vi "Autonomous Independent.vi"   [LabVIEW 2011]
doc: "This VI is called when autonomous begins, and will automatically be terminated when autonomous ends. You can carry out timed or sensor driven robot movement independently without needing to return to the caller."
uses:
  Robot Global Data.vi
types:
  T1 = typedef "WPI_MotorControlDeviceRef.ctl" = cluster{"DeviceStatus":errorcluster, "Type":enum16{"PWM", "CAN"}, "PWM":cluster{"Digital Module":T2, "PWM Channel":T3, "DeadBand":T4}, "CAN":cluster{"Device Number":u8, "Control Mode":T5, "Semaphore":T6, "Max Vout":dbl}, "Invert":bool, "TransformRef":T7, "InvTransformRef":T7}
  T2 = typedef "FPGA_TypedefDigitalModule.ctl" = enum16{"Digital Module 1", "Digital Module 2"}
  T3 = typedef "FPGA_DIOPWMChannel.ctl" = enum8{"PWM 1", "PWM 2", "PWM 3", "PWM 4", "PWM 5", "PWM 6", "PWM 7", "PWM 8", "PWM 9", "PWM 10", "Invalid"}
  T4 = typedef "WPI_PWMDeadband.ctl" = cluster{"Name":string, "maxPositivePwm":i32, "minPositivePwm":i32, "centerPwm":i32, "maxNegativePwm":i32, "minNegativePwm":i32, "angularRange":u16}
  T5 = typedef "WPI_CANJaguar_ControlMode.ctl" = enum8{"Percent VBus", "Current", "Speed", "Position", "Voltage"}
  T6 = typedef "Semaphore RefNum" = refnum<k1>
  T7 = typedef "WPI_PWMTransform_ConPane.ctl" = refnum<vi>
  T8 = typedef "WPI_ServoDeviceRef.ctl" = cluster{"DeviceStatus":errorcluster, "Digital Module":T2, "PWM Channel":T3, "DeadBand":T4}
  T9 = typedef "WPI_EncoderDevRef.ctl" = cluster{"DevStatus":errorcluster, "EncoderIndex":T10, "CounterIndex":T11, "DistancePerCount":dbl, "Decoding Type":T12}
  T10 = typedef "FPGA_EncoderIdx.ctl" = enum8{"Enc 0", "Enc 1", "Enc 2", "Enc 3", "Invalid"}
  T11 = typedef "FPGA_CounterCtrSystemIndex.ctl" = enum8{"Ctr 0", "Ctr 1", "Ctr 2", "Ctr 3", "Ctr 4", "Ctr 5", "Ctr 6", "Ctr 7", "Invalid"}
  T12 = typedef "WPI_EncoderType.ctl" = enum16{"1x", "2x", "4x"}
  T13 = typedef "WPI_GyroDevRef.ctl" = cluster{"DevStatus":errorcluster, "Analog Module":T14, "Analog Channel":T15, "Offset":dbl, "Gain (VoltsPerDegree/Second)":dbl}
  T14 = typedef "FPGA_TypedefAnalogModule.ctl" = enum16{"Analog Module 1", "Analog Module 2"}
  T15 = typedef "FPGA_AIChannel.ctl" = enum8{"AI 1", "AI 2", "AI 3", "AI 4", "AI 5", "AI 6", "AI 7", "AI 8", "Invalid"}
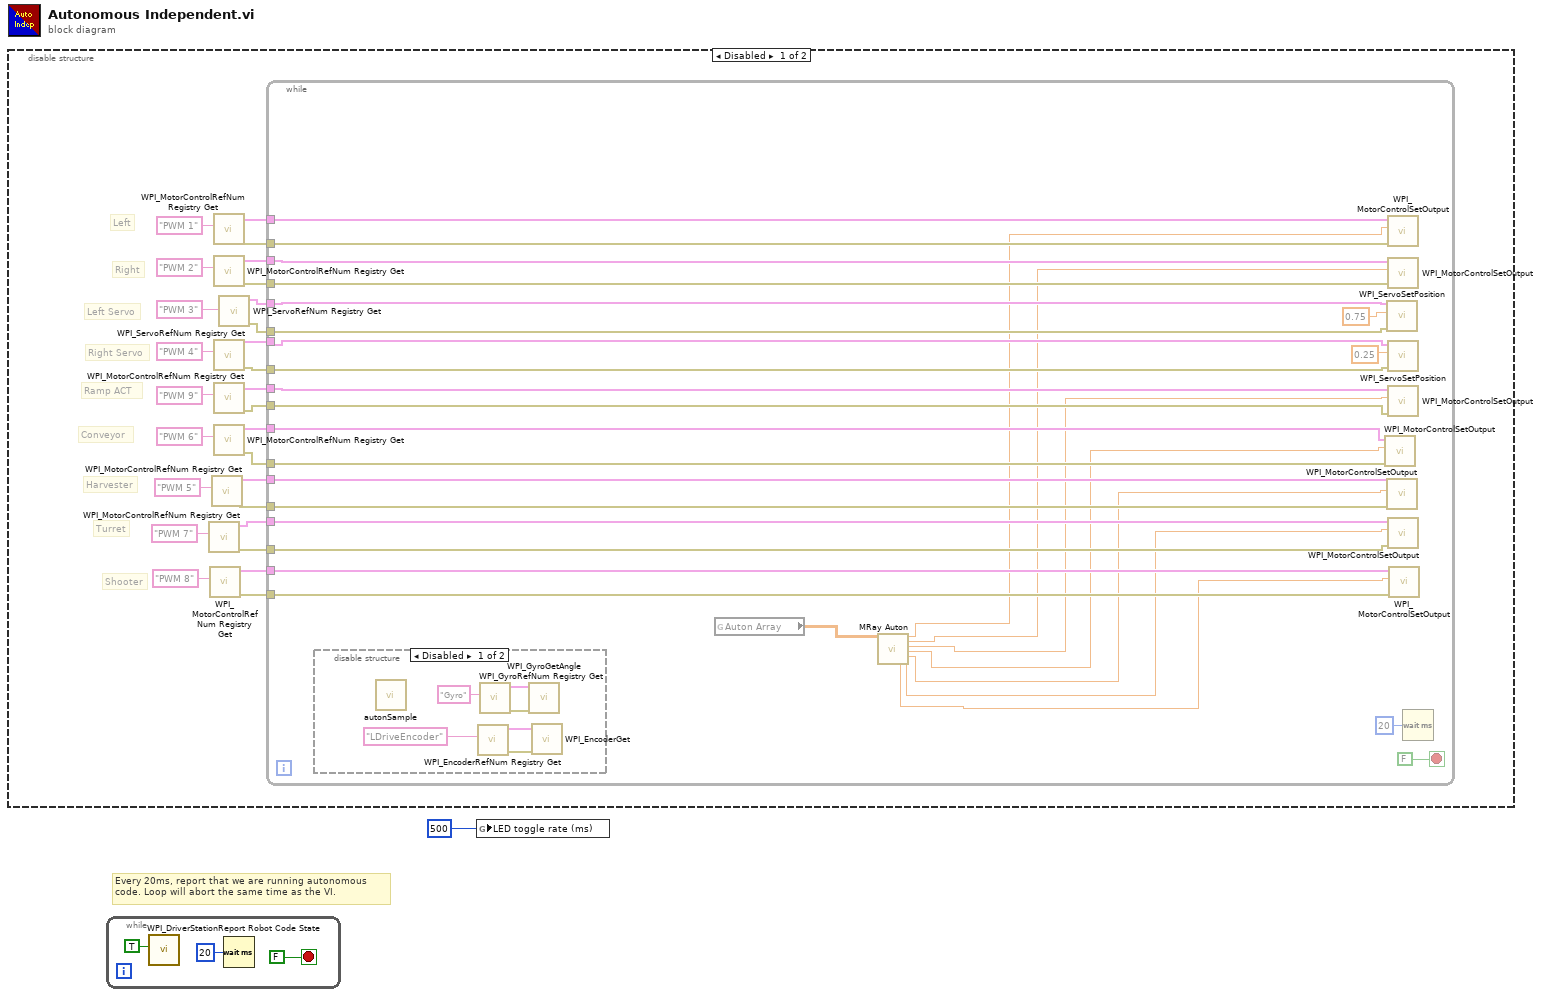
[diagram p0: block diagram]
diagram:
  # "Every 20ms, report that we are running autonomous\ncode. Loop will abort the same time as the VI."
  n1 = disable-structure shown="Disabled" {
    frame Disabled {
      # "Shooter"
      # "Turret"
      # "Conveyor"
      # "Harvester"
      # "Ramp ACT"
      # "Right Servo"
      # "Left Servo"
      # "Right"
      # "Left"
      n2 = call <vilib>:"WPI_MotorControlRefNum Registry Get.vi"("refnum name"="PWM 7") -> ("error out"=w9:errorcluster, "MotorControlDevRef"=w10:T1)  [unwired: 9 in]
      n3 = call <vilib>:"WPI_MotorControlRefNum Registry Get.vi"("refnum name"="PWM 8") -> ("error out"=w7:errorcluster, "MotorControlDevRef"=w8:T1)  [unwired: 9 in]
      n4 = call <vilib>:"WPI_MotorControlRefNum Registry Get.vi"("refnum name"="PWM 5") -> ("error out"=w11:errorcluster, "MotorControlDevRef"=w12:T1)  [unwired: 9 in]
      n5 = call <vilib>:"WPI_MotorControlRefNum Registry Get.vi"("refnum name"="PWM 1") -> ("error out"=w2:errorcluster, "MotorControlDevRef"=w24:T1)  [unwired: 9 in]
      n6 = call <vilib>:"WPI_MotorControlRefNum Registry Get.vi"("refnum name"="PWM 2") -> ("error out"=w3:errorcluster, "MotorControlDevRef"=w23:T1)  [unwired: 9 in]
      n7 = call <vilib>:"WPI_ServoRefNum Registry Get.vi"("refnum name"="PWM 4") -> ("error out"=w5:errorcluster, "ServoDeviceRef"=w22:T8)  [unwired: 9 in]
      n8 = call <vilib>:"WPI_MotorControlRefNum Registry Get.vi"("refnum name"="PWM 9") -> ("error out"=w6:errorcluster, "MotorControlDevRef"=w21:T1)  [unwired: 9 in]
      n9 = call <vilib>:"WPI_MotorControlRefNum Registry Get.vi"("refnum name"="PWM 6") -> ("error out"=w16:errorcluster, "MotorControlDevRef"=w17:T1)  [unwired: 9 in]
      n10 = call <vilib>:"WPI_ServoRefNum Registry Get.vi"("refnum name"="PWM 3") -> ("error out"=w4:errorcluster, "ServoDeviceRef"=w19:T8)  [unwired: 9 in]
      n11 = while {
        tunnel: w24 -> [w56]
        tunnel: w23 -> [w55]
        tunnel: w19 -> [w50]
        tunnel: w22 -> [w51]
        tunnel: w21 -> [w54]
        tunnel: w17 -> [w49]
        tunnel: w16 -> [w48]
        tunnel: w12 -> [w47]
        tunnel: w11 -> [w46]
        tunnel: w10 -> [w45]
        tunnel: w9 -> [w44]
        tunnel: w8 -> [w43]
        tunnel: w7 -> [w42]
        tunnel: w6 -> [w41]
        tunnel: w5 -> [w40]
        tunnel: w4 -> [w39]
        tunnel: w3 -> [w38]
        tunnel: w2 -> [w37]
        stop <- FALSE stop-if-true
        n12 = disable-structure shown="Disabled" {
          frame Disabled {
            n13 = call "autonSample.vi"() -> ()  [unwired: 9 in, 7 out]
            n14 = call <vilib>:"WPI_EncoderRefNum Registry Get.vi"("refnum name"="LDriveEncoder") -> ("error out"=w62:errorcluster, "EncoderDevRef"=w63:T9)  [unwired: 9 in]
            n15 = call <vilib>:"WPI_GyroRefNum Registry Get.vi"("refnum name"="Gyro") -> ("error out"=w60:errorcluster, "GyroDevRef"=w61:T13)  [unwired: 9 in]
            n16 = call <vilib>:"WPI_GyroGetAngle.vi"("error in (no error)"=w60, "GyroDevRef"=w61) -> ()  [unwired: 6 in, 4 out]
            n17 = call <vilib>:"WPI_EncoderGet.vi"("error in (no error)"=w62, "EncoderDevRef"=w63) -> ()  [unwired: 4 in, 6 out]
          }
          frame Enabled {
          }
        }
        n18 = global read "Robot Global Data.vi" "Auton Array"() -> (w36:dbl[][])
        n19 = call "MRay Auton.vi"("Auton Array"=w36) -> ("Shooter"=w29:dbl, "Left Drive"=w35:dbl, "Right Drive"=w34:dbl, "Ramp ACT motor"=w33:dbl, "Conveyor"=w32:dbl, "Harvester"=w31:dbl, "Turret Rotation"=w30:dbl)  [unwired: 12 in]
        n20 = call <vilib>:"WPI_MotorControlSetOutput.vi"("error in (no error)"=w48, "Output"=w32, "MotorControlDevRef"=w49) -> ()  [unwired: 7 in, 2 out]
        n21 = call <vilib>:"WPI_ServoSetPosition.vi"("error in (no error)"=w39, "Position"=0.75 ("Output"), "ServoDeviceRef"=w50) -> ()  [unwired: 7 in, 2 out]
        n22 = call <vilib>:"WPI_MotorControlSetOutput.vi"("error in (no error)"=w46, "Output"=w31, "MotorControlDevRef"=w47) -> ()  [unwired: 7 in, 2 out]
        n23 = call <vilib>:"WPI_MotorControlSetOutput.vi"("error in (no error)"=w37, "Output"=w35, "MotorControlDevRef"=w56) -> ()  [unwired: 7 in, 2 out]
        n24 = call <vilib>:"WPI_MotorControlSetOutput.vi"("error in (no error)"=w38, "Output"=w34, "MotorControlDevRef"=w55) -> ()  [unwired: 7 in, 2 out]
        n25 = call <vilib>:"WPI_ServoSetPosition.vi"("error in (no error)"=w40, "Position"=0.25 ("Output"), "ServoDeviceRef"=w51) -> ()  [unwired: 7 in, 2 out]
        n26 = call <vilib>:"WPI_MotorControlSetOutput.vi"("error in (no error)"=w41, "Output"=w33, "MotorControlDevRef"=w54) -> ()  [unwired: 7 in, 2 out]
        n27 = call <vilib>:"WPI_MotorControlSetOutput.vi"("error in (no error)"=w44, "Output"=w30, "MotorControlDevRef"=w45) -> ()  [unwired: 7 in, 2 out]
        n28 = call <vilib>:"WPI_MotorControlSetOutput.vi"("error in (no error)"=w42, "Output"=w29, "MotorControlDevRef"=w43) -> ()  [unwired: 7 in, 2 out]
        n29 = Wait (ms)(milliseconds to wait=u32 20) -> ()  [unwired: 1 out]
      }
    }
    frame Enabled {
    }
  }
  n30 = while {
    stop <- FALSE stop-if-true
    n31 = call <vilib>:"WPI_DriverStationReport Robot Code State.vi"("Autonomous"=TRUE) -> ()  [unwired: 10 in, 1 out]
    n32 = Wait (ms)(milliseconds to wait=u32 20) -> ()  [unwired: 1 out]
  }
  n33 = global write "Robot Global Data.vi" "LED toggle rate (ms)"(u32 500 ("LED ms toggle rate")) -> ()
